vi "5.0-Global.vi"() -> ()   [LabVIEW 2010]
uses:
  6-OCU Neurons/6.1-UDP Saitek.ctl
  6-OCU Neurons/MainControls.ctl
  6-OCU Neurons/MDF Array LatLong.ctl
  6-OCU Neurons/MDF LatLong.ctl
  6-OCU Neurons/MainIndicators.ctl
  4-High Neurons/4.2-Where Sensor Typedef.ctl
  4-High Neurons/Current GPS Data.ctl
  3-Midbrain/3.2-Where/_typedefs/3.2.1-VectorNav Data.ctl
  4-High Neurons/4.3-What Sensor Typedef.ctl
  3-Midbrain/3.3-What/_typedefs/3.3.1-LIDAR Data Typedef.ctl
  5.4 How/_TypeDefs/5.4-Clean How Sensor Typedef.ctl
  4-High Neurons/4.4-How Sensor Typedef.ctl
  4-High Neurons/4.0-Midbrain State.ctl
  6-OCU Neurons/6.0-Forbrain State.ctl
  4-High Neurons/4.1-Act Control Typedef.ctl
  4-High Neurons/4.1.0-Datatype Typedef.ctl
  6-OCU Neurons/MDF XY.ctl
panel:
  in  "Tab for Conveinience":T1(tab)
  in  "5.6.4 Act Control GUI":T2
  in  "5.6.4 Act Control":T2
  in  "5.6 Saitek Controler":T4 {"Right" scale=-32767.0..32767.0; "Left" scale=-32767.0..32767.0; "Yaw" scale=-32767.0..32767.0; "Roll" scale=-32767.0..32767.0; "Pitch" scale=-32767.0..32767.0}
  out "5.6.3 Forebrain Act Command":dbl[](array[numeric])
  in  "5.6.2 Act Command -  From Waypoint":dbl[](array[numeric])
  in  "5.1.2 MDF to Neo-Cortex":T5[](array[typedef]) {"X (waypoint)" format="%#_8g"; "Y  (waypoint)" format="%#_8g"}
  in  "5.1.1 MDF GPS":T6[](array[typedef]) {"Latitude (waypoint)" format="%#_8g"; "Longitude  (waypoint)" format="%#_8g"}
  in  "5.1.4 Where Data to Neo-Cortex":T7
  out "GPS Origin":T8 {"Longitude (dd.mmmmmm)" format="%#.6g"; "Lattitude (dd.mmmmmm)" format="%#.6g"}
  out "5.1.0 Where Check Light":bool
  in  "5.1.5 Current Waypoint":i32
  out "5.1.3 Where Am I?  Sensor":T9 {"4.2.2- Current GPS Data"."Longitude (dd.mmmmmm)" format="%#.6g"; "4.2.2- Current GPS Data"."Lattitude (dd.mmmmmm)" format="%#.6g"}
  in  "5.3.1-What's Around Me? Sensor":T12
  out "5.2.0 What Check Light":bool
  in  "5.4 Clean How Am I? Sensor":T14
  in  "5.4.4 How Am I? Sensor":T15
  in  "5.3.2 Mission Start Time":dbl
  out "5.3.0 How Check Light":bool
  out "5.3.1 MissionTime":dbl(knob) scale=0.0..10.0
  out "5.5 Hypo Check Light":bool
  out "5.5 Hpo T - Act Out":cluster{"Motor1":i16, "Motor 2":i16}
  in  "5.5 How?Forebrain":cluster{"Motor1":i16, "Motor 2":i16}
  in  "5.7.2 Main Indicators":T17 {"5.3.1 MissionTimeAuto" scale=0.0..10.0; "4.2-Where Am I? Sensor"."4.2.2- Current GPS Data"."Longitude (dd.mmmmmm)" format="%#.6g"; "4.2-Where Am I? Sensor"."4.2.2- Current GPS Data"."Lattitude (dd.mmmmmm)" format="%#.6g"}
  in  "5.7.1 Main Controls":T18 {"5.1.1 MDF GPS 2"."Latitude (waypoint)" format="%#_8g"; "5.1.1 MDF GPS 2"."Longitude  (waypoint)" format="%#_8g"; "6.1-Saitek Controller"."Right" scale=-32767.0..32767.0; "6.1-Saitek Controller"."Left" scale=-32767.0..32767.0; "6.1-Saitek Controller"."Yaw" scale=-32767.0..32767.0; "6.1-Saitek Controller"."Roll" scale=-32767.0..32767.0; "6.1-Saitek Controller"."Pitch" scale=-32767.0..32767.0}
  in  "6.0 Forebrain State":T20
  in  "5.8 Begin":bool
  out "Stop Loops":bool
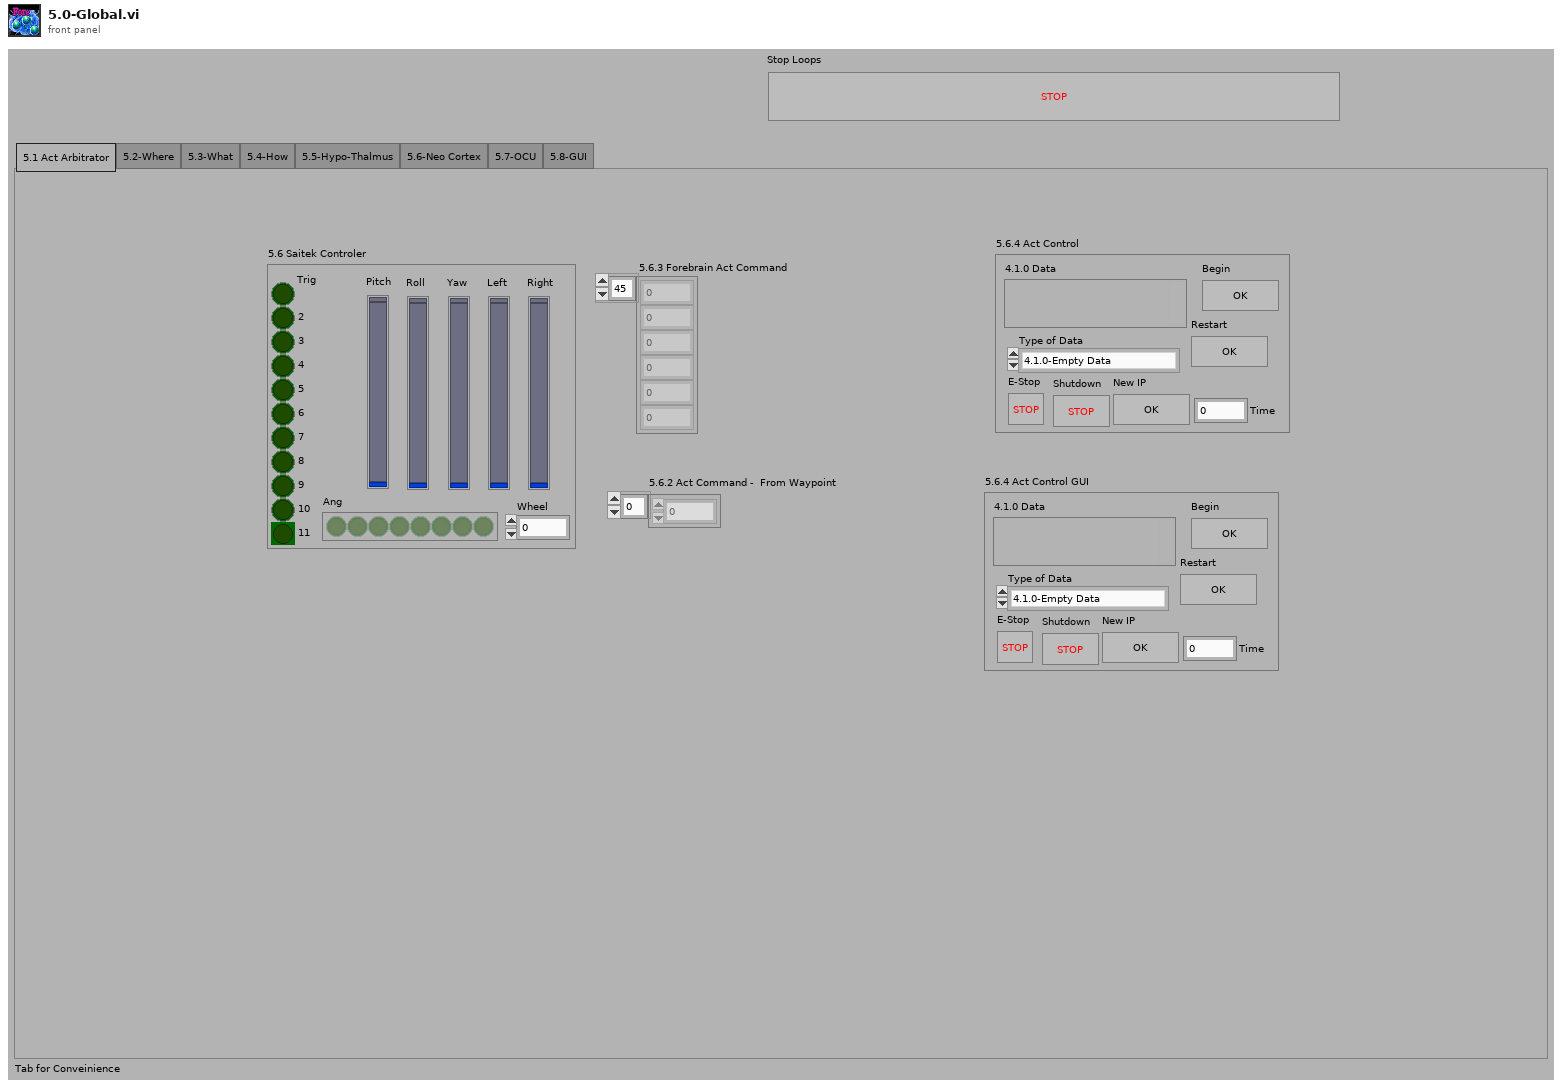
[diagram p1: front panel]
types:
  T1 = enum32{"5.1 Act Arbitrator", "5.2-Where", "5.3-What", "5.4-How", "5.5-Hypo-Thalmus", "5.6-Neo Cortex", "5.7-OCU", "5.8-GUI"}
  T2 = typedef "4.1-Act Control Typedef.ctl" = cluster{"4.1.0 Data":variant, "Type of Data":T3, "E-Stop":bool, "Restart":bool, "New IP":bool, "Begin":bool, "Time":i32, "Shutdown":bool}
  T3 = typedef "4.1.0-Datatype Typedef.ctl" = enum16{"4.1.0-Empty Data", "4.1.1-Joystick Data", "4.1.2-Behavioral Data"}
  T4 = typedef "6.1-UDP Saitek.ctl" = cluster{"Trig":bool, "2":bool, "3":bool, "4":bool, "5":bool, "6":bool, "7":bool, "8":bool, "9":bool, "10":bool, "11":bool, "Pitch":i32, "Ang":bool[], "Wheel":dbl, "Roll":i32, "Yaw":i32, "Left":i32, "Right":i32}
  T5 = typedef "MDF XY.ctl" = cluster{"Waypoint #":dbl, "X (waypoint)":ext, "Y  (waypoint)":ext, "Vel (desired)":dbl, "Dwell Time":dbl, "Behavior":enum16{"OpenFieldTransit", "WallFollow", "LaneFollow", "ManualMode"}, "Expand1":dbl, "Expand2":dbl, "Expand3":dbl}
  T6 = typedef "MDF LatLong.ctl" = cluster{"Waypoint #":dbl, "Latitude (waypoint)":ext, "Longitude  (waypoint)":ext, "Vel (desired)":dbl, "Dwell Time":dbl, "Behavior":enum16{"OpenFieldTransit", "WallFollow", "LaneFollow", "ManualMode"}, "Expand1":dbl, "Expand2":dbl, "Expand3":dbl}
  T7 = cluster{"X (Current)":dbl, "Y (Current) ":dbl, "Heading":dbl, "Steering Angle":dbl}
  T8 = cluster{"Lattitude (dd.mmmmmm)":ext, "Longitude (dd.mmmmmm)":ext}
  T9 = typedef "4.2-Where Sensor Typedef.ctl" = cluster{"4.2.2- Current GPS Data":T10, "4.2.1-VectorNav Data":T11, "4.2.1-VectorNav Status":string}
  T10 = typedef "Current GPS Data.ctl" = cluster{"Lattitude (dd.mmmmmm)":ext, "Longitude (dd.mmmmmm)":ext, "EST Time":timestamp}
  T11 = typedef "3.2.1-VectorNav Data.ctl" = cluster{"Yaw":dbl, "Pitch":dbl, "Roll":dbl}
  T12 = typedef "4.3-What Sensor Typedef.ctl" = cluster{"LIDAR Data":T13}
  T13 = typedef "3.3.1-LIDAR Data Typedef.ctl" = cluster{"Angle array":dbl[], "Magnitude array ":dbl[]}
  T14 = typedef "5.4-Clean How Sensor Typedef.ctl" = cluster{"Motor Speed Integer":i32, "Drive Position Integer":i32, "Lidar Position Integer":i32, "Lidar Motor Position Integer":i32, "Steering Position Integer":i32, "Battery Voltage Fxp":dbl, "Drive Encoder Cable Check":bool, "Lidar Drive Encoder Cable Check":bool, "Steer Encoder Cable Check":bool, "Lidar Pos Encoder Cable Check":bool, "Mod Buttons & Blinky Cable Check":bool, "Lidar Data Cable Check":bool, "Drive Motor Cable Check":bool, "Vector Nav Cable Check":bool, "Lidar Drive Cable Check":bool, "Steer Drive Cable Check":bool, "Reverse?":bool, "2.1  Steering Control Voltage":dbl, "2.1 Drive Control Voltage":dbl, "2.1  Lidar Control Voltage":dbl, "2.5.7 A*B":dbl, "2.1  Steering PID Output":dbl, "2.1 Drive PID Output":dbl, "2.1  Lidar PID Output":dbl, "2.1.1 Drive Error":dbl, "2.1.1 Drive Error I":dbl, "2.1.1 Drive Error D":dbl, "2.1.2 Steering Error":dbl, "2.1.2 Steering Error I":dbl, "2.1.2 Steering Error D":dbl, "2.1.3 Lidar Error":dbl, "2.1.3 Lidar Error I":dbl, "2.1.3 Lidar Error D":dbl, "VectorNav Ack Query":bool, "VectorNav Read Byte":u8, "VectorNav Read Status":enum16{"Waiting", "Reading", "Done"}}
  T15 = typedef "4.4-How Sensor Typedef.ctl" = cluster{"Motor Speed Integer":i32, "Drive Position Integer":i32, "Lidar Position Integer":i32, "Lidar Motor Position Integer":i32, "Steering Position Integer":i32, "Battery Voltage Fxp":dbl, "Drive Encoder Cable Check":bool, "Lidar Drive Encoder Cable Check":bool, "Steer Encoder Cable Check":bool, "Lidar Pos Encoder Cable Check":bool, "Mod Buttons & Blinky Cable Check":bool, "Lidar Data Cable Check":bool, "Drive Motor Cable Check":bool, "Vector Nav Cable Check":bool, "Lidar Drive Cable Check":bool, "Steer Drive Cable Check":bool, "Reverse?":bool, "2.1  Steering Control Voltage":dbl, "2.1 Drive Control Voltage":dbl, "2.1  Lidar Control Voltage":dbl, "2.5.7 A*B":dbl, "2.1  Steering PID Output":dbl, "2.1 Drive PID Output":dbl, "2.1  Lidar PID Output":dbl, "2.1.1 Drive Error":dbl, "2.1.1 Drive Error I":dbl, "2.1.1 Drive Error D":dbl, "2.1.2 Steering Error":dbl, "2.1.2 Steering Error I":dbl, "2.1.2 Steering Error D":dbl, "2.1.3 Lidar Error":dbl, "2.1.3 Lidar Error I":dbl, "2.1.3 Lidar Error D":dbl, "VectorNav Ack Query":bool, "VectorNav Read Byte":u8, "VectorNav Read Status":enum16{"Waiting", "Reading", "Done"}, "4.0-Midbrain State":T16}
  T16 = typedef "4.0-Midbrain State.ctl" = enum16{"Startup", "Waiting to Run", "Running-OlinOval", "Running-ChannelFollow", "Running-WallFollow", "Running-OpenTransit", "Running-Joystick Training", "Shutdown", "Restart", "New IP"}
  T17 = typedef "MainIndicators.ctl" = cluster{"Where?":bool, "What?":bool, "4.2-Where Am I? Sensor":T9, "4.3-What's Around Me? Sensor":T12, "5.3.1 MissionTimeAuto":dbl, "5.4 Clean How Am I? Sensor":T14, "How?":bool}
  T18 = typedef "MainControls.ctl" = cluster{"6.1-Saitek Controller":T4, "Manual Override":bool, "5.1.1 MDF GPS 2":T19}
  T19 = typedef "MDF Array LatLong.ctl" = T6[]
  T20 = typedef "6.0-Forbrain State.ctl" = enum16{"Startup", "Waiting to Run", "Running-OlinOval", "Running-ChannelFollow", "Running-WallFollow", "Running-OpenTransit", "Running-Joystick Training", "Shutdown", "Restart", "New IP"}
diagram:
